vi "New From Context.vi"(8 "error in (no error)":errorcluster, 11 "Search Context":T1) -> (0 "error out":errorcluster, 3 "Search out":refnum<class "Search.lvclass">)   [LabVIEW 2020, in "Better Search.lvlib" / "Search.lvclass"]
uses:
  Search.lvclass
  Data Types/Search Context.ctl
  Data Types/Start Search Type.ctl
  Data Types/Type Reflection Item.ctl
  Search Result/Search Result.lvclass
  Search.lvclass/Search.ctl
  Better Search.lvlib
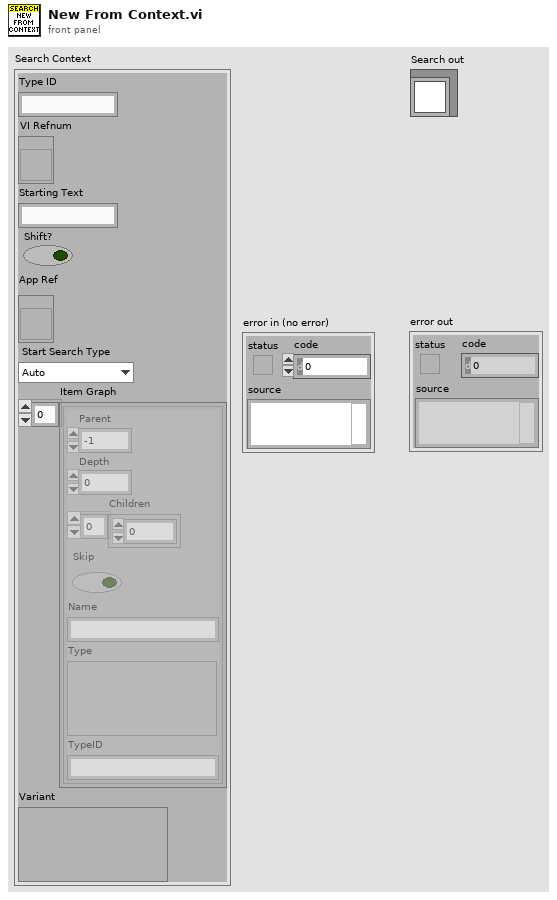
[diagram p1: front panel]
types:
  T1 = typedef "Better Search.lvlib/Search Context.ctl" = cluster{"Type ID":string, "VI Refnum":refnum<vi>, "Starting Text":string, "Shift?":bool, "App Ref":refnum<vi>, "Start Search Type":T2, "Item Graph":T3[], "Variant":variant}
  T2 = typedef "Better Search.lvlib/Start Search Type.ctl" = enum16{"Auto", "Text", "Data Type", "Bundle"}
  T3 = typedef "Better Search.lvlib/Type Reflection Item.ctl" = cluster{"Parent":i32, "Depth":i32, "Children":i32[], "Skip":bool, "Name":string, "Type":variant, "TypeID":string}
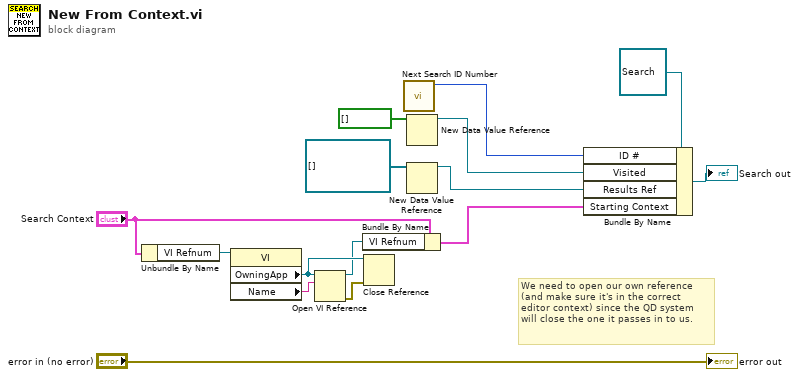
[diagram p0: block diagram]
diagram:
  # "We need to open our own reference (and make sure it's in the correct editor context) since the QD system will close the one it passes in to us."
  n1 = Unbundle By Name("Search Context") -> ("VI Refnum"=w9:refnum<vi>)
  n2 = property class="VI"(reference=w9) -> ("OwningApp"=w10:refnum<vi>, "Name"=w12:string)  [unwired: 1 in, 2 out]
  n3 = Open VI Reference(application reference (local)=w10, vi path=w12) -> (vi reference=w7:refnum<vi>, error out=w11:errorcluster)  [unwired: 4 in]
  n4 = Bundle By Name(cluster="Search Context", "VI Refnum"=w7) -> (w6:T1)
  n5 = Close Reference(reference=w10, error in (no error)=w11) -> ()  [unwired: 1 out]
  n6 = call "Next Search ID Number.vi"() -> ("Next ID #"=w1:i32)  [unwired: 11 in]
  n7 = New Data Value Reference(data value=bool[] []) -> (data value reference=w2:refnum<data-value>)  [unwired: 1 in, 1 out]
  n8 = New Data Value Reference(data value=refnum<class "Search Result.lvclass">[] []) -> (data value reference=w4:refnum<data-value>)  [unwired: 1 in, 1 out]
  n9 = Bundle By Name(cluster=refnum<class "Search.lvclass"> refnum ("Search in"), "ID #"=w1, "Visited"=w2, "Results Ref"=w4, "Starting Context"=w6) -> (→"Search out":refnum<class "Search.lvclass">)
  "error out" <- "error in (no error)"
